vi "Controller.vi"(8 "error in (no error)":errorcluster) -> (0 "error out":errorcluster)   [LabVIEW 2017]
uses:
  Type Definitions/Queue FG Options.ctl
panel:
  in  "stop":bool
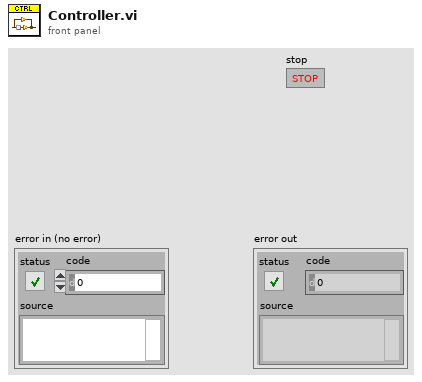
[diagram p1: front panel]
types:
  T1 = typedef "Queue FG Options.ctl" = enum16{"Set", "Get", "Read", "Write"}
  T2 = typedef "Controller Message.ctl" = cluster{"Message Info":T3, "Message Data":variant}
  T3 = typedef "Controller States.ctl" = enum16{"Initial", "Login", "Idle", "Balance Inquiry", "Deposit", "Withdrawal", "Fast Cash", "Terminate", "Shutdown"}
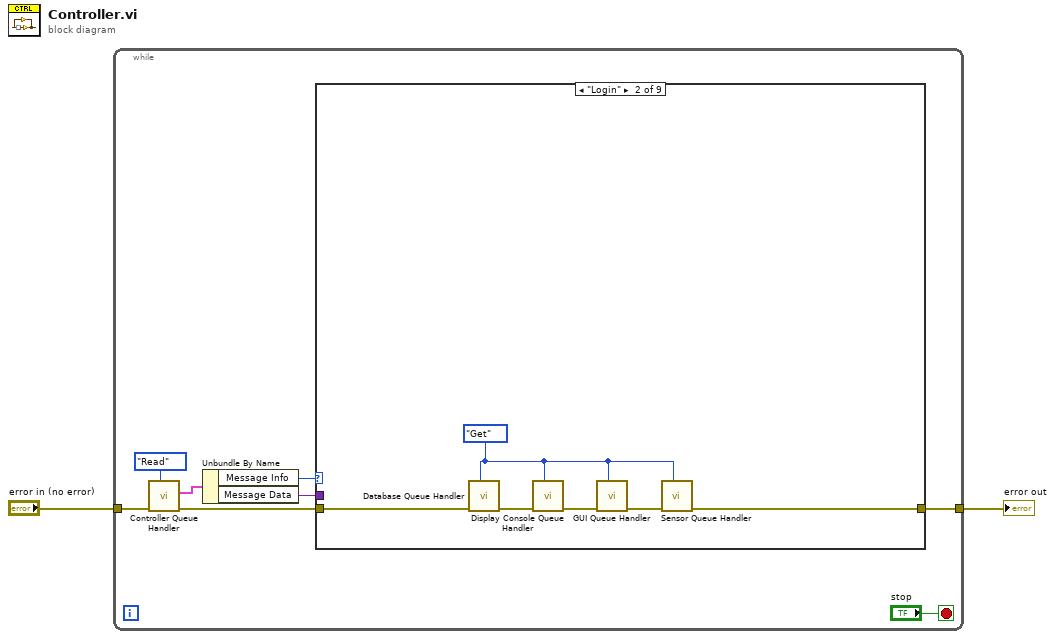
[diagram p0: block diagram]
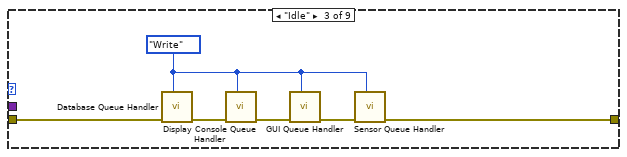
[diagram p3: hidden frame]
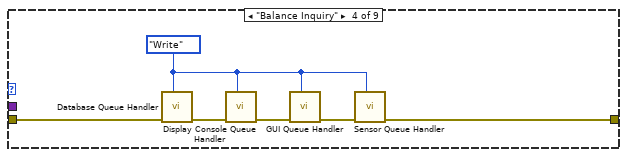
[diagram p4: hidden frame]
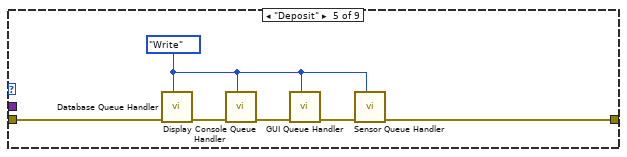
[diagram p5: hidden frame]
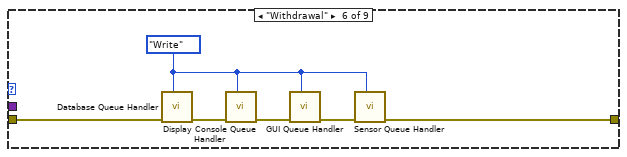
[diagram p6: hidden frame]
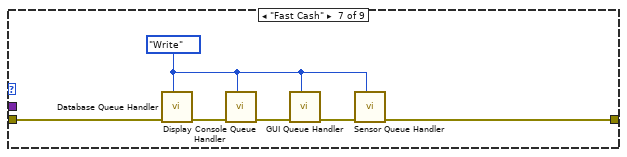
[diagram p7: hidden frame]
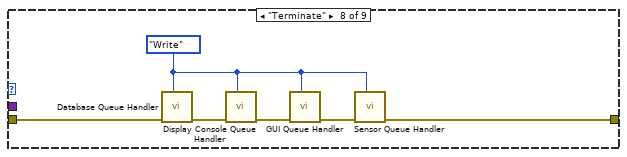
[diagram p8: hidden frame]
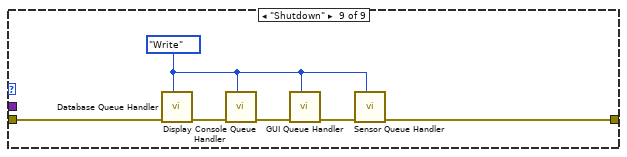
[diagram p9: hidden frame]
diagram:
  n1 = while {
    tunnel: "error in (no error)" -> [w8]
    tunnel: [w3] -> w1
    stop <- "stop" stop-if-true
    n2 = call "Controller Queue Handler.vi"("Action"=Queue_FG_Options."Read", "error in (no error)"=w8) -> ("error out"=w4:errorcluster, "Message out"=w7:T2)  [unwired: 7 in, 1 out]
    n3 = Unbundle By Name(w7) -> ("Message Info"=w6:T3, "Message Data"=w5:variant)
    n4 = case shown="\"Login\"" w6 {
      tunnel: w5 -> [_ _ _ _ _ _ _ _ _]
      tunnel: w4 -> [w11 w17 w23 w29 w35 w41 w47 w53 w59]
      tunnel: [w11 w15 w21 w27 w33 w39 w45 w51 w57] -> w3
      frame "Initial", Default {
      }
      frame "Login" {
        w12 = Queue_FG_Options."Get" ("Action")
        n5 = call "Database Queue Handler.vi"("Action"=w12, "error in (no error)"=w17) -> ("error out"=w16:errorcluster)  [unwired: 7 in, 2 out]
        n6 = call "Display Console Queue Handler.vi"("Action"=w12, "error in (no error)"=w16) -> ("error out"=w14:errorcluster)  [unwired: 7 in, 2 out]
        n7 = call "GUI Queue Handler.vi"("Action"=w12, "error in (no error)"=w14) -> ("error out"=w13:errorcluster)  [unwired: 6 in, 3 out]
        n8 = call "Sensor Queue Handler.vi"("Action"=w12, "error in (no error)"=w13) -> ("error out"=w15:errorcluster)  [unwired: 6 in, 3 out]
      }
      frame "Idle" {
        w18 = Queue_FG_Options."Write" ("Action")
        n9 = call "Database Queue Handler.vi"("Action"=w18, "error in (no error)"=w23) -> ("error out"=w22:errorcluster)  [unwired: 7 in, 2 out]
        n10 = call "Display Console Queue Handler.vi"("Action"=w18, "error in (no error)"=w22) -> ("error out"=w20:errorcluster)  [unwired: 7 in, 2 out]
        n11 = call "GUI Queue Handler.vi"("Action"=w18, "error in (no error)"=w20) -> ("error out"=w19:errorcluster)  [unwired: 6 in, 3 out]
        n12 = call "Sensor Queue Handler.vi"("Action"=w18, "error in (no error)"=w19) -> ("error out"=w21:errorcluster)  [unwired: 6 in, 3 out]
      }
      frame "Balance Inquiry" {
        w24 = Queue_FG_Options."Write" ("Action")
        n13 = call "Database Queue Handler.vi"("Action"=w24, "error in (no error)"=w29) -> ("error out"=w28:errorcluster)  [unwired: 7 in, 2 out]
        n14 = call "Display Console Queue Handler.vi"("Action"=w24, "error in (no error)"=w28) -> ("error out"=w26:errorcluster)  [unwired: 7 in, 2 out]
        n15 = call "GUI Queue Handler.vi"("Action"=w24, "error in (no error)"=w26) -> ("error out"=w25:errorcluster)  [unwired: 6 in, 3 out]
        n16 = call "Sensor Queue Handler.vi"("Action"=w24, "error in (no error)"=w25) -> ("error out"=w27:errorcluster)  [unwired: 6 in, 3 out]
      }
      frame "Deposit" {
        w30 = Queue_FG_Options."Write" ("Action")
        n17 = call "Database Queue Handler.vi"("Action"=w30, "error in (no error)"=w35) -> ("error out"=w34:errorcluster)  [unwired: 7 in, 2 out]
        n18 = call "Display Console Queue Handler.vi"("Action"=w30, "error in (no error)"=w34) -> ("error out"=w32:errorcluster)  [unwired: 7 in, 2 out]
        n19 = call "GUI Queue Handler.vi"("Action"=w30, "error in (no error)"=w32) -> ("error out"=w31:errorcluster)  [unwired: 6 in, 3 out]
        n20 = call "Sensor Queue Handler.vi"("Action"=w30, "error in (no error)"=w31) -> ("error out"=w33:errorcluster)  [unwired: 6 in, 3 out]
      }
      frame "Withdrawal" {
        w36 = Queue_FG_Options."Write" ("Action")
        n21 = call "Database Queue Handler.vi"("Action"=w36, "error in (no error)"=w41) -> ("error out"=w40:errorcluster)  [unwired: 7 in, 2 out]
        n22 = call "Display Console Queue Handler.vi"("Action"=w36, "error in (no error)"=w40) -> ("error out"=w38:errorcluster)  [unwired: 7 in, 2 out]
        n23 = call "GUI Queue Handler.vi"("Action"=w36, "error in (no error)"=w38) -> ("error out"=w37:errorcluster)  [unwired: 6 in, 3 out]
        n24 = call "Sensor Queue Handler.vi"("Action"=w36, "error in (no error)"=w37) -> ("error out"=w39:errorcluster)  [unwired: 6 in, 3 out]
      }
      frame "Fast Cash" {
        w42 = Queue_FG_Options."Write" ("Action")
        n25 = call "Database Queue Handler.vi"("Action"=w42, "error in (no error)"=w47) -> ("error out"=w46:errorcluster)  [unwired: 7 in, 2 out]
        n26 = call "Display Console Queue Handler.vi"("Action"=w42, "error in (no error)"=w46) -> ("error out"=w44:errorcluster)  [unwired: 7 in, 2 out]
        n27 = call "GUI Queue Handler.vi"("Action"=w42, "error in (no error)"=w44) -> ("error out"=w43:errorcluster)  [unwired: 6 in, 3 out]
        n28 = call "Sensor Queue Handler.vi"("Action"=w42, "error in (no error)"=w43) -> ("error out"=w45:errorcluster)  [unwired: 6 in, 3 out]
      }
      frame "Terminate" {
        w48 = Queue_FG_Options."Write" ("Action")
        n29 = call "Database Queue Handler.vi"("Action"=w48, "error in (no error)"=w53) -> ("error out"=w52:errorcluster)  [unwired: 7 in, 2 out]
        n30 = call "Display Console Queue Handler.vi"("Action"=w48, "error in (no error)"=w52) -> ("error out"=w50:errorcluster)  [unwired: 7 in, 2 out]
        n31 = call "GUI Queue Handler.vi"("Action"=w48, "error in (no error)"=w50) -> ("error out"=w49:errorcluster)  [unwired: 6 in, 3 out]
        n32 = call "Sensor Queue Handler.vi"("Action"=w48, "error in (no error)"=w49) -> ("error out"=w51:errorcluster)  [unwired: 6 in, 3 out]
      }
      frame "Shutdown" {
        w54 = Queue_FG_Options."Write" ("Action")
        n33 = call "Database Queue Handler.vi"("Action"=w54, "error in (no error)"=w59) -> ("error out"=w58:errorcluster)  [unwired: 7 in, 2 out]
        n34 = call "Display Console Queue Handler.vi"("Action"=w54, "error in (no error)"=w58) -> ("error out"=w56:errorcluster)  [unwired: 7 in, 2 out]
        n35 = call "GUI Queue Handler.vi"("Action"=w54, "error in (no error)"=w56) -> ("error out"=w55:errorcluster)  [unwired: 6 in, 3 out]
        n36 = call "Sensor Queue Handler.vi"("Action"=w54, "error in (no error)"=w55) -> ("error out"=w57:errorcluster)  [unwired: 6 in, 3 out]
      }
    }
  }
  "error out" <- w1
